vi "Glob_Ref.vi"() -> ()   [LabVIEW 2019]
uses:
  _ctrl/Sinple-sequence-type.ctl
  Durability/sequence_single.ctl
  Durability/common/UI dev-operator.ctl
panel:
  in  "TrPos":dbl
  in  "simulation":bool
  in  "Oscilloscope_LCR":cluster{"Record Len":i32, "Time Div":u16}={"Record Len"=4, "Time Div"=0} {"Time Div" items=["10m", "20ms", "50ms", "100ms", "200ms", "500ms", "1s", "2s", "5s", "10s", "20s", "30s", "1min", "2min", "5min"]; "Record Len" items=["10k", "25k", "50k", "100k", "250k", "500k", "1M", "2.5M", "5M", "10M", "25M", "50M", "100M", "250M", "500M", "1G", "2G", "4G", "5G", "10G", "20G", "50G"]}
  in  "Control Signal_LCR":T1={"Freq"=50.0, "level[V]"=12.0, "duty"=50.0, "On time[ms]"=50.0}
  in  "Oscilloscope_HV":cluster{"Record Len":i32, "Time Div":u16}={"Record Len"=4, "Time Div"=0} {"Time Div" items=["10m", "20ms", "50ms", "100ms", "200ms", "500ms", "1s", "2s", "5s", "10s", "20s", "30s", "1min", "2min", "5min"]; "Record Len" items=["10k", "25k", "50k", "100k", "250k", "500k", "1M", "2.5M", "5M", "10M", "25M", "50M", "100M", "250M", "500M", "1G", "2G", "4G", "5G", "10G", "20G", "50G"]}
  in  "Control Signal_HV":T1={"Freq"=50.0, "level[V]"=12.0, "duty"=50.0, "On time[ms]"=50.0}
  in  "Oscilloscope_LV":cluster{"Record Len":i32, "Time Div":u16}={"Record Len"=4, "Time Div"=0} {"Time Div" items=["10m", "20ms", "50ms", "100ms", "200ms", "500ms", "1s", "2s", "5s", "10s", "20s", "30s", "1min", "2min", "5min"]; "Record Len" items=["10k", "25k", "50k", "100k", "250k", "500k", "1M", "2.5M", "5M", "10M", "25M", "50M", "100M", "250M", "500M", "1G", "2G", "4G", "5G", "10G", "20G", "50G"]}
  in  "Control Signal_LV":T1={"Freq"=50.0, "level[V]"=12.0, "duty"=50.0, "On time[ms]"=50.0}
  out "NumDiv_ResLV":dbl
  out "NumData_ResLV":dbl
  out "NumDiv_OHV":dbl
  out "NumData_OHV":dbl
  out "NumDiv_OLV":dbl
  out "NumData_OLV":dbl
  in  "DSP Selection":enum32{"DSP HV", "DSP LV"}(radio)
  out "Array_temp":T2(array[cluster])
  out "부하전압":dbl
  out "date/time_finish":string
  out "testState":T3
  in  "check_hw":bool
  out "t1":u32
  in  "start_seq":bool
  in  "stop":bool
  in  "Single sequence":T4=enum."RC"
  out "OverLoad":i32 caption="Query"
  out "checkCom":bool
  in  "Single seq data":cluster{"Sequence type":T5}
  out "NumDiv_b3":dbl
  out "NumData_b3":dbl
  out "NumDiv_b2":dbl
  out "NumData_b2":dbl
  out "NumDiv_b1":dbl
  out "NumData_b1":dbl
  in  "Oscilloscope_B1":cluster{"Record Len":i32, "Time Div":u16}={"Record Len"=4, "Time Div"=0} {"Time Div" items=["10m", "20ms", "50ms", "100ms", "200ms", "500ms", "1s", "2s", "5s", "10s", "20s", "30s", "1min", "2min", "5min"]; "Record Len" items=["10k", "25k", "50k", "100k", "250k", "500k", "1M", "2.5M", "5M", "10M", "25M", "50M", "100M", "250M", "500M", "1G", "2G", "4G", "5G", "10G", "20G", "50G"]}
  in  "Control Signal_B1":T1={"Freq"=50.0, "level[V]"=12.0, "duty"=50.0, "On time[ms]"=50.0}
  in  "Oscilloscope_rc":cluster{"Record Len":i32, "Time Div":u16}={"Record Len"=4, "Time Div"=0} {"Time Div" items=["10m", "20ms", "50ms", "100ms", "200ms", "500ms", "1s", "2s", "5s", "10s", "20s", "30s", "1min", "2min", "5min"]; "Record Len" items=["10k", "25k", "50k", "100k", "250k", "500k", "1M", "2.5M", "5M", "10M", "25M", "50M", "100M", "250M", "500M", "1G", "2G", "4G", "5G", "10G", "20G", "50G"]}
  in  "Control Signal_rc":T1={"Freq"=0.0, "level[V]"=0.0, "duty"=0.0, "On time[ms]"=50.0}
  out "NumDiv_rc":dbl
  out "NumData_rc":dbl
  in  "Oscilloscope_B3":cluster{"Record Len":i32, "Time Div":u16}={"Record Len"=4, "Time Div"=0} {"Time Div" items=["10m", "20ms", "50ms", "100ms", "200ms", "500ms", "1s", "2s", "5s", "10s", "20s", "30s", "1min", "2min", "5min"]; "Record Len" items=["10k", "25k", "50k", "100k", "250k", "500k", "1M", "2.5M", "5M", "10M", "25M", "50M", "100M", "250M", "500M", "1G", "2G", "4G", "5G", "10G", "20G", "50G"]}
  in  "Control Signal_B3":T1={"Freq"=50.0, "level[V]"=12.0, "duty"=50.0, "On time[ms]"=50.0}
  in  "Oscilloscope_B2":cluster{"Record Len":i32, "Time Div":u16}={"Record Len"=4, "Time Div"=0} {"Time Div" items=["10m", "20ms", "50ms", "100ms", "200ms", "500ms", "1s", "2s", "5s", "10s", "20s", "30s", "1min", "2min", "5min"]; "Record Len" items=["10k", "25k", "50k", "100k", "250k", "500k", "1M", "2.5M", "5M", "10M", "25M", "50M", "100M", "250M", "500M", "1G", "2G", "4G", "5G", "10G", "20G", "50G"]}
  in  "Control Signal_B2":T1={"Freq"=50.0, "level[V]"=12.0, "duty"=50.0, "On time[ms]"=50.0}
  out "NumDiv_res":dbl
  out "NumDatal_res":dbl
  in  "Oscilloscope_res":cluster{"Record Len":i32, "Time Div":u16}={"Record Len"=4, "Time Div"=0} {"Time Div" items=["10m", "20ms", "50ms", "100ms", "200ms", "500ms", "1s", "2s", "5s", "10s", "20s", "30s", "1min", "2min", "5min"]; "Record Len" items=["10k", "25k", "50k", "100k", "250k", "500k", "1M", "2.5M", "5M", "10M", "25M", "50M", "100M", "250M", "500M", "1G", "2G", "4G", "5G", "10G", "20G", "50G"]}
  in  "Control Signal_res":T1={"Freq"=0.0, "level[V]"=0.0, "duty"=0.0, "On time[ms]"=50.0}
  out "Curr_dsp":dbl
  out "Volt_dsp":dbl
  in  "table_raw":refnum<vi>
  in  "table_result":refnum<vi>
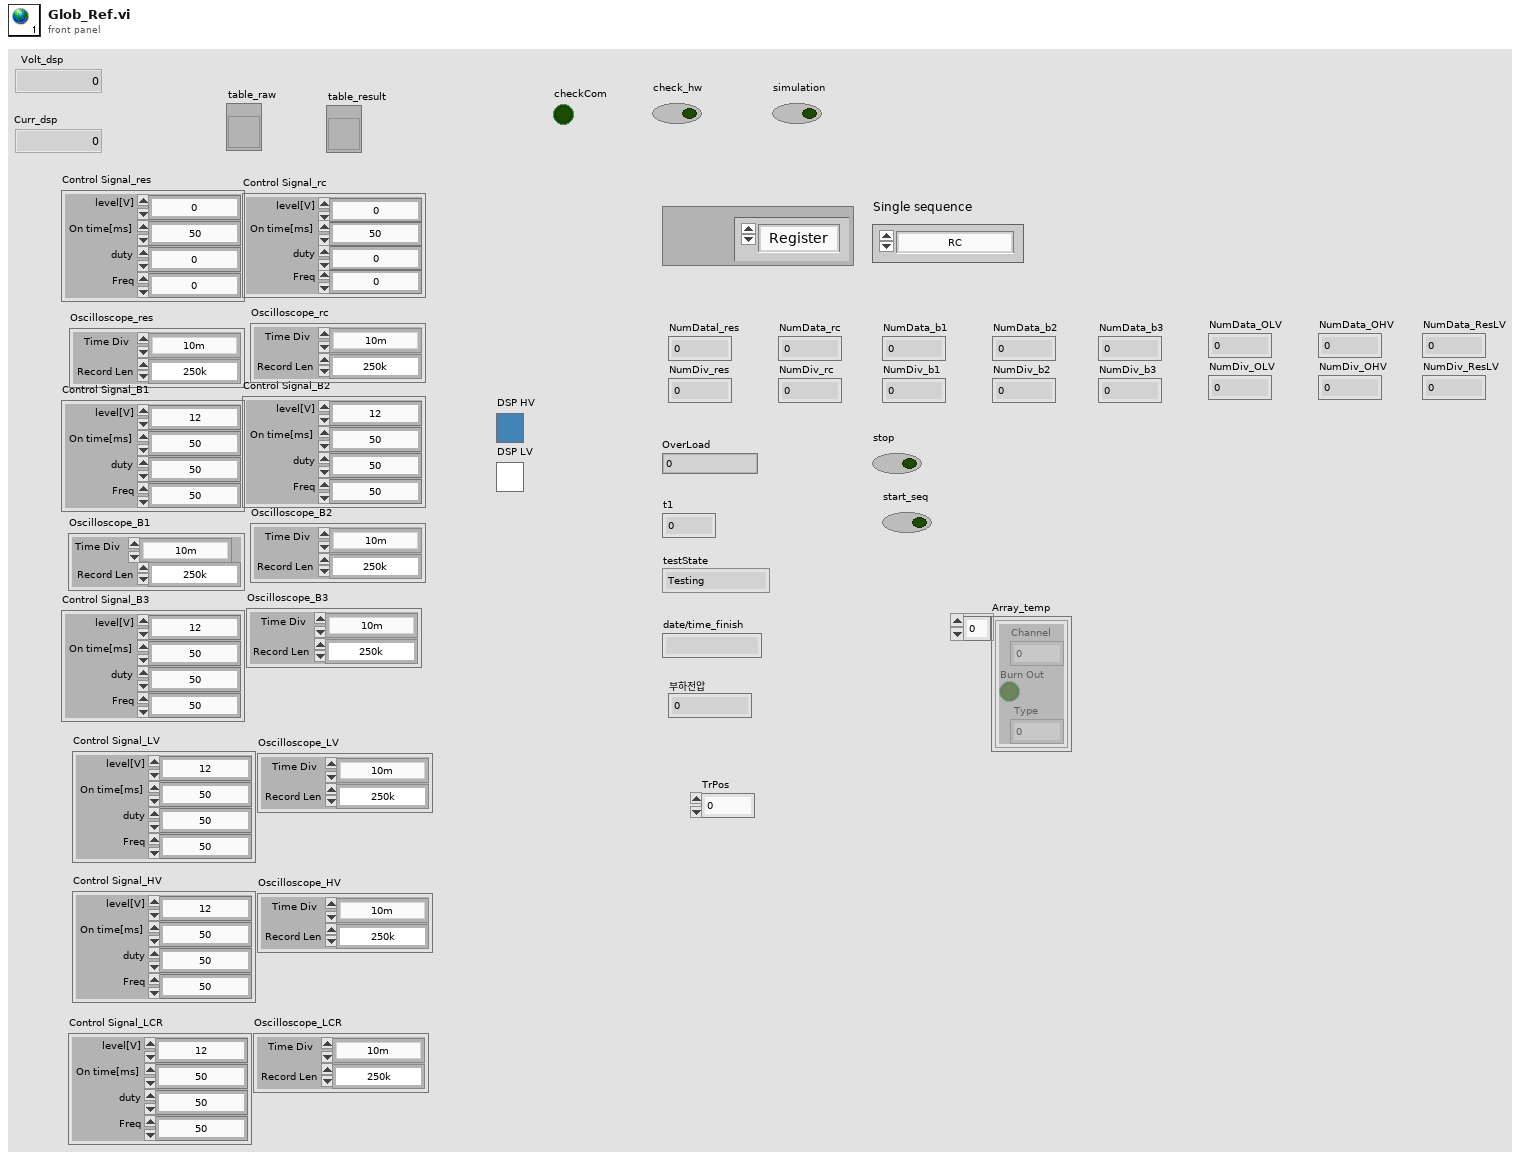
[diagram p1: front panel]
types:
  T1 = cluster{"Freq":dbl, "level[V]":dbl, "duty":dbl, "On time[ms]":dbl}
  T2 = cluster{"Channel":u16, "Burn Out":bool, " Type ":i32}[]
  T3 = typedef "UI dev-operator.ctl" = enum16{"Testing", "Admin", "Operator", "Finish", "Ready"}
  T4 = typedef "sequence_single.ctl" = enum16{"Register", "RC", "B1", "B2", "B3", "Oper_LV", "Oper_HV", "ContR_LV"}
  T5 = typedef "Sinple-sequence-type.ctl" = enum16{"Register", "RC", "B1", "B2", "B3"}
diagram:
